vi "tsdiag_can_request_transfer_exit.vi"(6 "AReqCase":i32, 7 "ADataSize":i32, 8 "error in (no error)":errorcluster, 9 "ASourceData":u8[](array[numeric]), 10 "ADiagModuleIndex":i32, 11 "路径输入":path) -> (0 "error out":errorcluster, 2 "return":i32, 3 "路径输出":path)   [LabVIEW 2014]
doc: "37服务，请求退出数据传输。"
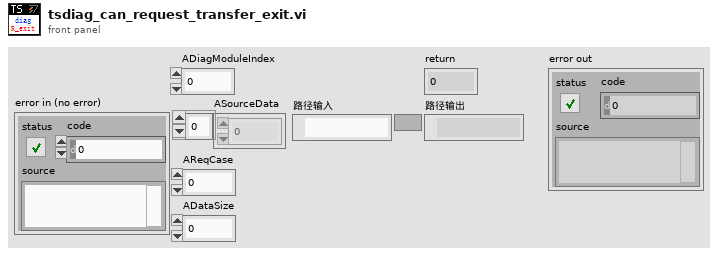
[diagram p1: front panel]
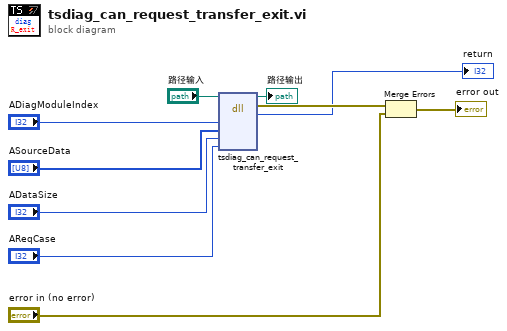
[diagram p0: block diagram]
diagram:
  n1 = dll-call lib="D:/Program Files (x86)/TOSUN/TSMaster/bin/TSMaster.dll" fn="tsdiag_can_request_transfer_exit"(path in="路径输入", "ADiagModuleIndex"="ADiagModuleIndex", "ASourceData"="ASourceData", "ADataSize"="ADataSize", "AReqCase"="AReqCase") -> (path out=→"路径输出":path, error out=w10:errorcluster, "ACode"=→"return":i32)  [unwired: 6 in]
  n2 = Merge Errors(w10, "error in (no error)") -> (→"error out":errorcluster)
